vi "buzzer (SubVI).vi"(7 "BuzzerOn":bool, 8 "Error In":errorcluster, 10 "Time Target (s)":dbl(slide)=0.5 scale=0.1..1.0, 11 "Digital Output in":refnum<class "Digital Output.lvclass">) -> (0 "Error Out":errorcluster, 3 "Digital Output out":refnum<class "Digital Output.lvclass">)   [LabVIEW 2020]
uses:
  <vilib>/CISH Robotics/L4VMX VMXpi/Digital Output/Digital Output.lvclass
panel:
  # "DO:18"
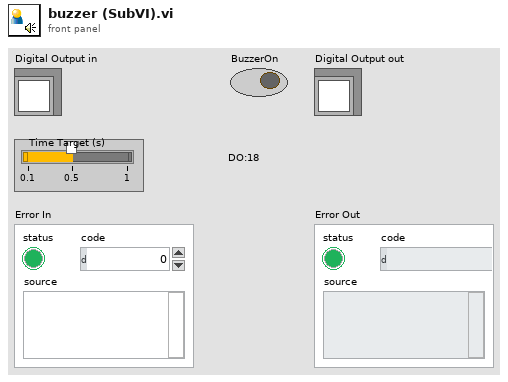
[diagram p1: front panel]
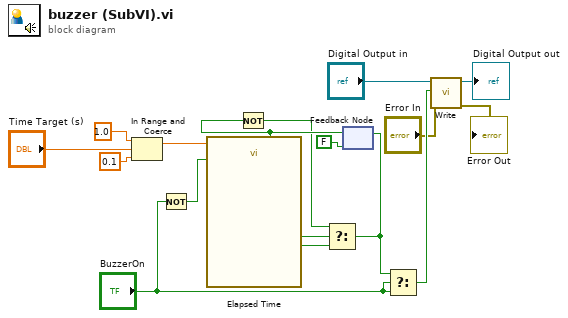
[diagram p0: block diagram]
diagram:
  n1 = In Range and Coerce(upper limit=1.0, x="Time Target (s)", lower limit=0.1) -> (coerced(x)=w3:dbl)  [unwired: 1 out]
  n2 = Not(x="BuzzerOn") -> (.not. x?=w13:bool)
  n3 = call "Elapsed Time"("Time Target (s)"=w3, "Reset"=w13) -> ("Time has Elapsed"=w9:bool)  [unwired: 10 in, 7 out]
  n4 = feedback #1(FALSE) -> (w12:bool)
  n5 = Not(x=w12) -> (.not. x?=w10:bool)
  n6 = Select(t=w10, s=w9, f=w12) -> (s? t:f=w14:bool)
  n7 = feedback-in #1(w14) -> ()
  n8 = Select(t=w14, s="BuzzerOn", f="BuzzerOn") -> (s? t:f=w15:bool)
  n9 = call <vilib>:"Write.vi"("Error In"="Error In", "Value"=w15, "Digital Output Object"="Digital Output in") -> ("Error Out"=→"Error Out":errorcluster, "Digital Output Object"=→"Digital Output out":refnum<class "Digital Output.lvclass">)  [unwired: 7 in]
